vi "simple.vi"() -> ()   [LabVIEW 2012]
uses:
  <userlib>/libximc/libximc.lvlib
panel:
  in  "WND 1":i32=1 min=1 max=8
  in  "WND 2":i32=1 min=1 max=8
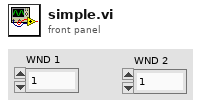
[diagram p1: front panel]
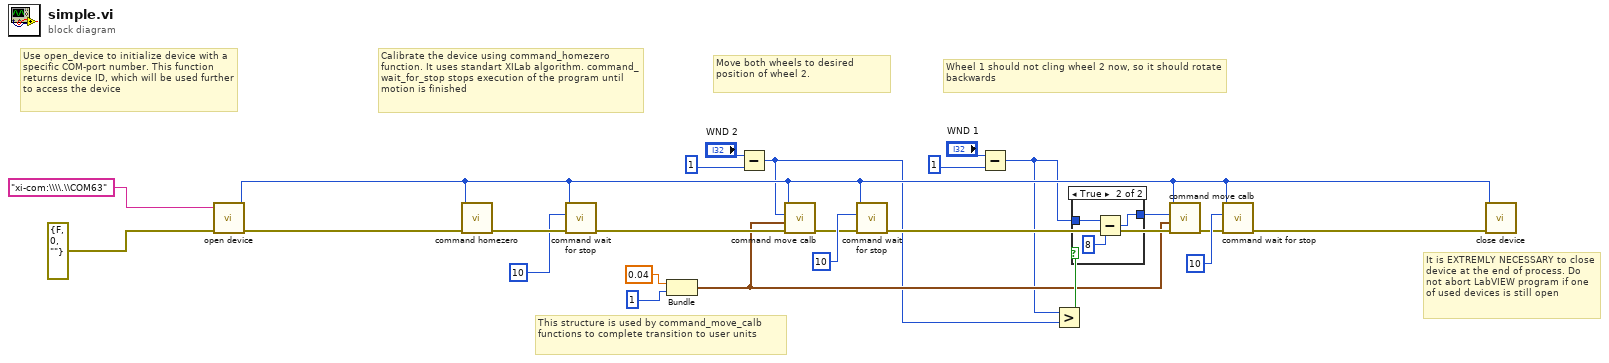
[diagram p0: block diagram]
diagram:
  # "It is EXTREMLY NECESSARY to close device at the end of process. Do not abort LabVIEW program if one of used devices is still open"
  # "Wheel 1 should not cling wheel 2 now, so it should rotate backwards"
  # "Move both wheels to desired position of wheel 2."
  # "This structure is used by command_move_calb functions to complete transition to user units"
  # "Calibrate the device using command_homezero function. It uses standart XILab algorithm. command_wait_for_stop stops execution of the program until motion is finished"
  # "Use open_device to initialize device with a specific COM-port number. This function returns device ID, which will be used further to access the device"
  n1 = call <userlib>:"open device.vi"("error in (no error)"=errorcluster {"status"=FALSE, "code"=0, "source"=""}, "uri"="xi-com:\\\\.\\COM63") -> ("error out"=w22:errorcluster, "function return"=w7:i32)  [unwired: 8 in]
  n2 = call <userlib>:"command homezero.vi"("error in (no error)"=w22, "id"=w7) -> ("error out"=w21:errorcluster)  [unwired: 8 in, 1 out]
  n3 = call <userlib>:"command wait for stop.vi"("error in (no error)"=w21, "refresh_interval_ms"=10, "id"=w7) -> ("error out"=w15:errorcluster)  [unwired: 7 in, 1 out]
  n4 = Bundle(0.04, 1) -> (w9:cluster{dbl, i32})  [unwired: 1 in]
  n5 = Subtract(x="WND 2", y=1) -> (x-y=w6:i32)
  n6 = call <userlib>:"command move calb.vi"("error in (no error)"=w15, "calibration"=w9, "Position"=w6, "id"=w7) -> ("error out"=w17:errorcluster)  [unwired: 6 in, 1 out]
  n7 = call <userlib>:"command wait for stop.vi"("error in (no error)"=w17, "refresh_interval_ms"=10, "id"=w7) -> ("error out"=w12:errorcluster)  [unwired: 7 in, 1 out]
  n8 = Subtract(x="WND 1", y=1) -> (x-y=w3:i32)
  n9 = Greater?(x=w3, y=w6) -> (0:w14:bool)
  n10 = case shown="True" w14 {
    tunnel: w3 -> [w25 w27]
    tunnel: [w25 w26] -> w11
    frame False {
    }
    frame True {
      n11 = Subtract(x=w27, y=8) -> (x-y=w26:i32)
    }
  }
  n12 = call <userlib>:"command move calb.vi"("error in (no error)"=w12, "calibration"=w9, "Position"=w11, "id"=w7) -> ("error out"=w10:errorcluster)  [unwired: 6 in, 1 out]
  n13 = call <userlib>:"command wait for stop.vi"("error in (no error)"=w10, "refresh_interval_ms"=10, "id"=w7) -> ("error out"=w8:errorcluster)  [unwired: 7 in, 1 out]
  n14 = call <userlib>:"close device.vi"("error in (no error)"=w8, "id"=w7) -> ()  [unwired: 7 in, 3 out]
